vi "Factorial_calculator.vi"(0 "M":i64, 5 "N":i64, 9 "Operations":T1(ring), 11 "Stop":bool) -> (4 "C":i64)   [LabVIEW 2021]
doc: "This VI calculates the value for the following operations with operand as M and N.\na. Factorial of M+N\nb. Sum of factorials of first M natural numbers\nc. Sum of factorials of first N whole numbers\nd. Greater of M and N"
panel:
  # "CALCULATE THE OUTPUT 'C'"
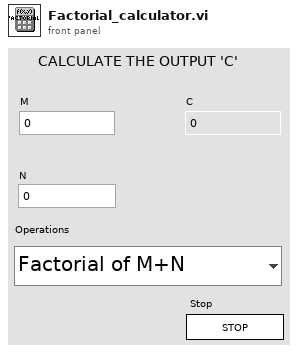
[diagram p1: front panel]
types:
  T1 = enum16{"Factorial of M+N", "Sum of factorials of first M natural numbers", "Sum of factorials of first N whole number", "Greater of M and N"}
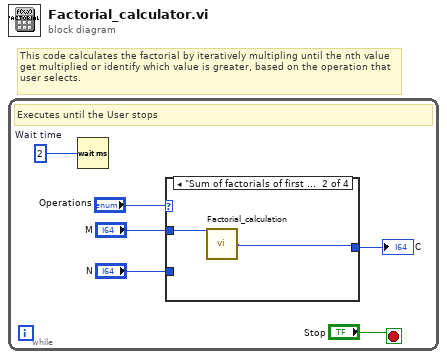
[diagram p0: block diagram]
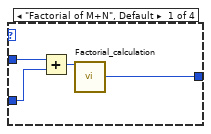
[diagram p2: hidden frame]
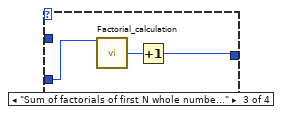
[diagram p3: hidden frame]
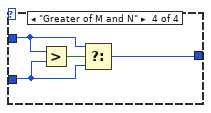
[diagram p4: hidden frame]
diagram:
  # "This code calculates the factorial by iteratively multipling until the nth value get multiplied or identify which value is greater, based on the operation that user selects."
  n1 = while {
    stop <- "Stop" stop-if-true
    w1 = u32 2  # Wait time
    # "Executes until the User stops"
    n2 = Wait (ms)(milliseconds to wait=w1) -> ()  [unwired: 1 out]
    n3 = case shown="\"Sum of factorials of first M natural numbers\"" "Operations" {
      tunnel: "M" -> [w10 w12 _ w17]
      tunnel: "N" -> [w9 _ w14 w16]
      tunnel: [w7 w11 w13 w19] -> w2
      frame "Factorial of M+N", Default {
        n4 = Add(x=w10, y=w9) -> (x+y=w8:i64)
        n5 = call "Factorial_calculation.vi"("n"=w8) -> ("Factorial of n"=w7:i64)  [unwired: 13 in, 1 out]
      }
      frame "Sum of factorials of first M natural numbers" {
        n6 = call "Factorial_calculation.vi"("n"=w12) -> ("Sum of Factorials  of first n Numbers"=w11:i64)  [unwired: 13 in, 1 out]
      }
      frame "Sum of factorials of first N whole number" {
        n7 = call "Factorial_calculation.vi"("n"=w14) -> ("Sum of Factorials  of first n Numbers"=w15:i64)  [unwired: 13 in, 1 out]
        n8 = Increment(x=w15) -> (x+1=w13:i64)
      }
      frame "Greater of M and N" {
        n9 = Greater?(x=w17, y=w16) -> (0:w18:bool)
        n10 = Select(t=w17, s=w18, f=w16) -> (s? t:f=w19:i64)
      }
    }
    "C" <- w2
  }
